vi "readInXml.vi"(8 "error in (no error)":errorcluster, 10 "Path":path, 11 "PixelflySettings in":refnum<class "PixelflySettings.lvclass">) -> (0 "error out":errorcluster, 3 "PixelflySettings out":refnum<class "PixelflySettings.lvclass">)   [LabVIEW 2009, in "Tools.lvlib" / "Settings.lvlib" / "PixelflySettings.lvclass"]
uses:
  PixelflySettings.lvclass
  NativeXML/NativeXML.lvclass
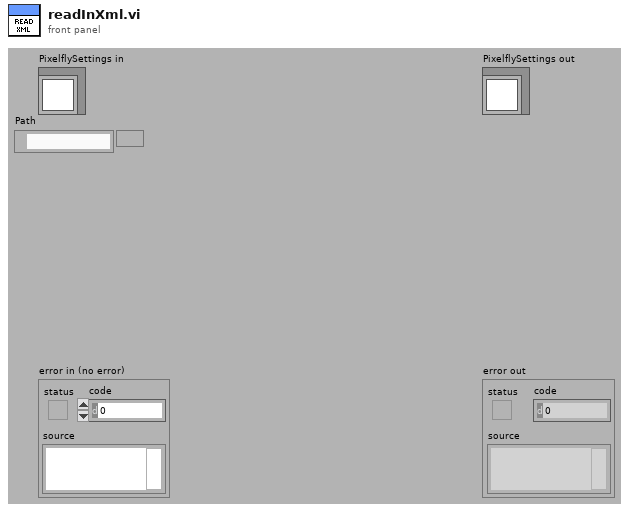
[diagram p1: front panel]
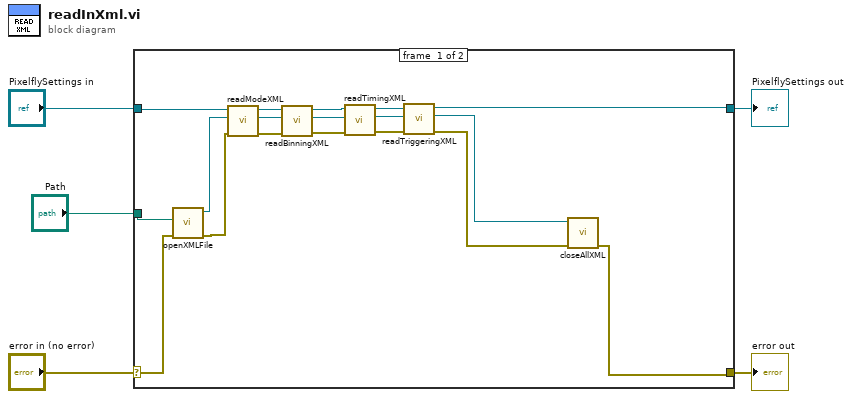
[diagram p0: block diagram]
diagram:
  n1 = case shown="No Error" "error in (no error)" {
    selector: "error in (no error)" -> [w22 w25]
    tunnel: [w6 w25] -> w4
    tunnel: [w9 w24] -> w2
    tunnel: "PixelflySettings in" -> [w21 w24]
    tunnel: "Path" -> [w23 _]
    frame #0 {
      n2 = call "openXMLFile.vi"("error in (no error)"=w22, "Path"=w23) -> ("error out"=w19:errorcluster, "NativeXML out"=w20:refnum<class "NativeXML.lvclass">)  [unwired: 8 in]
      n3 = call "readModeXML.vi"("error in (no error)"=w19, "NativeXML in"=w20, "PixelflySettings in"=w21) -> ("error out"=w16:errorcluster, "NativeXML out"=w17:refnum<class "NativeXML.lvclass">, "PixelflySettings out"=w18:refnum<class "PixelflySettings.lvclass">)  [unwired: 6 in]
      n4 = call "readBinningXML.vi"("error in (no error)"=w16, "NativeXML in"=w17, "PixelflySettings in"=w18) -> ("error out"=w14:errorcluster, "NativeXML out"=w13:refnum<class "NativeXML.lvclass">, "PixelflySettings out"=w15:refnum<class "PixelflySettings.lvclass">)  [unwired: 6 in]
      n5 = call "readTimingXML.vi"("error in (no error)"=w14, "NativeXML in"=w13, "PixelflySettings in"=w15) -> ("error out"=w11:errorcluster, "NativeXML out"=w10:refnum<class "NativeXML.lvclass">, "PixelflySettings out"=w12:refnum<class "PixelflySettings.lvclass">)  [unwired: 6 in]
      n6 = call "readTriggeringXML.vi"("error in (no error)"=w11, "NativeXML in"=w10, "PixelflySettings in"=w12) -> ("error out"=w7:errorcluster, "NativeXML out"=w8:refnum<class "NativeXML.lvclass">, "PixelflySettings out"=w9:refnum<class "PixelflySettings.lvclass">)  [unwired: 6 in]
      n7 = call "closeAllXML.vi"("error in (no error)"=w7, "NativeXML in"=w8) -> ("error out"=w6:errorcluster)  [unwired: 9 in]
    }
    frame #1 {
    }
  }
  "error out" <- w4
  "PixelflySettings out" <- w2
